vi "device log.vi"(10 "new element/subarray":string, 11 "worker ID":i32) -> ()   [LabVIEW 2020]
uses:
  status/item name.vi
  <vilib>/Utility/file.llb/Write Delimited Spreadsheet (string).vi
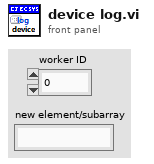
[diagram p1: front panel]
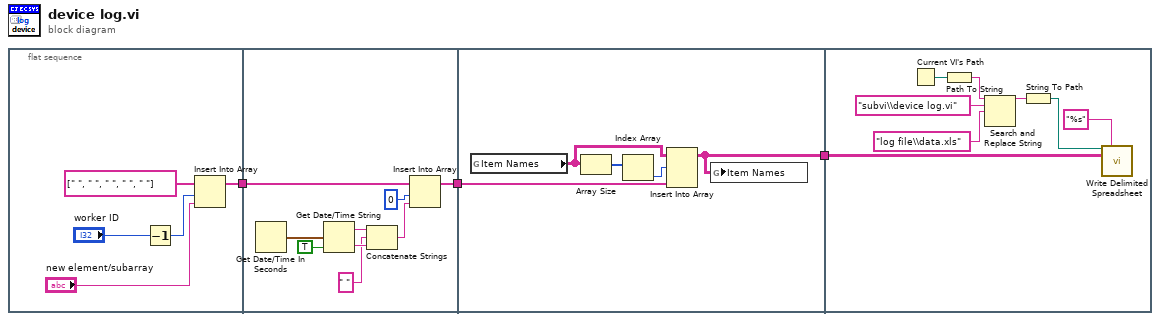
[diagram p0: block diagram]
diagram:
  n1 = flat-sequence {
    tunnel: [w7] -> w3
    tunnel: w3 -> [w11]
    tunnel: [w10] -> w2
    tunnel: w2 -> [w20]
    tunnel: [w18] -> w1
    tunnel: w1 -> [w30]
    frame #0 {
      n2 = Decrement(x="worker ID") -> (x-1=w4:i32)
      n3 = Insert Into Array(array=string[] [" ", " ", " ", " ", " "], index=w4, new element="new element/subarray") -> (w7:string[])
    }
    frame #1 {
      n4 = Get Date/Time In Seconds() -> (seconds since 1Jan1904=w15:timestamp)
      n5 = Get Date/Time String(seconds (now)=w15, want seconds? (F)=TRUE) -> (date string=w16:string, time string=w17:string)  [unwired: 1 in]
      n6 = Concatenate Strings(w16, " " ("string"), w17) -> (w14:string)
      n7 = Insert Into Array(array=w11, index=0, new element=w14) -> (w10:string[])
    }
    frame #2 {
      n8 = global read "item name.vi" "Item Names"() -> (w19:string[][])
      n9 = Array Size(array=w19) -> (size(s)=w22:i32[])
      n10 = Index Array(array=w22) -> (element=w21:i32)  [unwired: 1 in]
      n11 = Insert Into Array(array=w19, index (row)=w21, new element=w20) -> (w18:string[][])  [unwired: 1 in]
      n12 = global write "item name.vi" "Item Names"(w18) -> ()
    }
    frame #3 {
      n13 = Current VI's Path() -> (path=w26:path)
      n14 = Path To String(path=w26) -> (string=w27:string)
      n15 = Search and Replace String(input string=w27, search string="subvi\\device log.vi", replace string="log file\\data.xls" ("substring (\"\")")) -> (result string=w28:string)  [unwired: 5 in, 3 out]
      n16 = String To Path(string=w28) -> (path=w23:path)
      n17 = call-poly <vilib>:"Write Delimited Spreadsheet.vi"("file path (dialog if empty)"=w23, "format (%s)"="%s", "2D data"=w30) -> ()  [unwired: 11 in, 2 out]
    }
  }
